vi "half_wave_selection_array.vi"(6 "signal in":waveform(dbl), 9 "data":waveform(dbl), 10 "Numeric":dbl, 11 "frequency":dbl) -> (1 "waveform out":waveform(dbl), 2 "waveform out 2":waveform(dbl), 3 "waveform out 3":waveform(dbl))   [LabVIEW 2017]
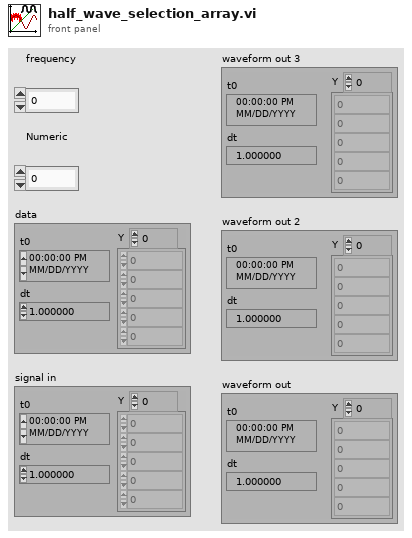
[diagram p1: front panel]
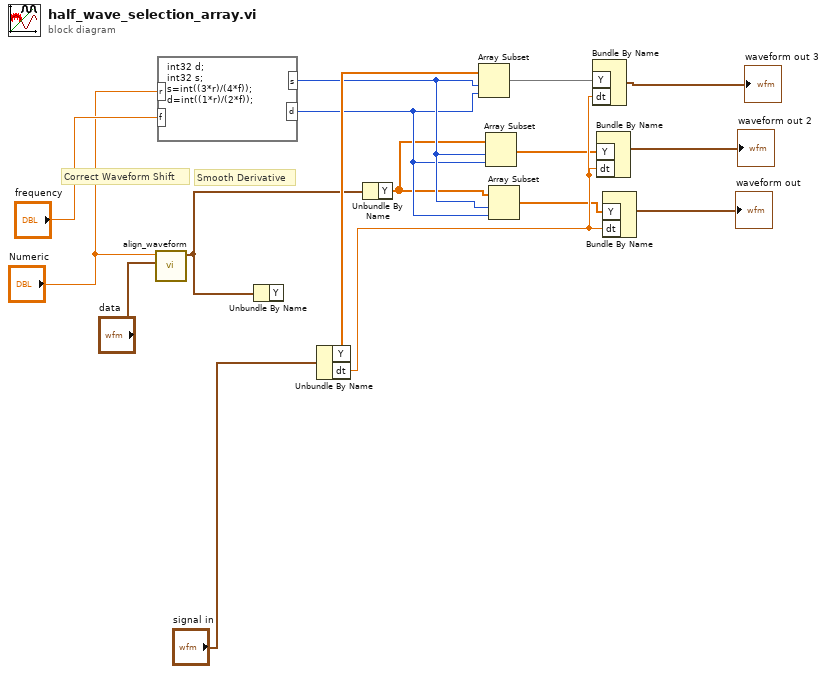
[diagram p0: block diagram]
diagram:
  # "Smooth Derivative"
  # "Correct Waveform Shift"
  n1 = call "align_waveform.vi"("Input Waveform"="data", "Sample Rate to be Wired"="Numeric") -> ("Output Waveform"=w4:waveform(dbl))  [unwired: 9 in]
  n2 = formula code="int32 d;\nint32 s;\ns=int((3*r)/(4*f));\nd=int((1*r)/(2*f));"("f"="frequency", "r"="Numeric") -> ("d"=w5:i32, "s"=w6:i32)
  n3 = Unbundle By Name(w4) -> ()  [unwired: 1 out]
  n4 = Unbundle By Name("signal in") -> ("Y"=w8:dbl[], "dt"=w9:dbl)
  n5 = Unbundle By Name(w4) -> ("Y"=w2:dbl[])
  n6 = Array Subset(array=w8, index=w6, length=w5) -> (w7:dbl[])
  n7 = Array Subset(array=w2, index=w6, length=w5) -> (w1:dbl[])
  n8 = Array Subset(array=w2, index=w6, length=w5) -> (w3:dbl[])
  n9 = Bundle By Name("Y"=w7, "dt"=w9) -> (→"waveform out 3":waveform(dbl))  [unwired: 1 in]
  n10 = Bundle By Name("Y"=w1, "dt"=w9) -> (→"waveform out 2":waveform(dbl))  [unwired: 1 in]
  n11 = Bundle By Name("Y"=w3, "dt"=w9) -> (→"waveform out":waveform(dbl))  [unwired: 1 in]
